vi "Convert Rx Config (4 Channels).vi"(0 "rx config":T2={"transfer mode"=enum."Finite", "sample rate"=10000000.0, "number of samples"=8192, "start trigger"=enum."Immediate", "daughterboard 0 config"={"rf enable 0"=TRUE, "rf config 0"={"antenna"="RX1", "frequency"=2000000000.0, "gain"=40.0}, "rf enable 1"=TRUE, "rf config 1"={"antenna"="RX2", "frequency"=2000000000.0, "gain"=40.0}, "lo configuration"=enum."Independent"}, "daughterboard 1 config"={"rf enable 2"=TRUE, "rf config 2"={"antenna"="RX1", "frequency"=2000000000.0, "gain"=40.0}, "rf enable 3"=TRUE, "rf config 3"={"antenna"="RX2", "frequency"=2000000000.0, "gain"=40.0}, "lo configuration"=enum."Independent"}} {"daughterboard 1 config"."rf config 3"."gain" format="%#.1f"; "daughterboard 1 config"."rf config 3"."frequency" format="%#.3pHz"; "daughterboard 1 config"."rf config 2"."gain" format="%#.1f"; "daughterboard 1 config"."rf config 2"."frequency" format="%#.3pHz"; "daughterboard 0 config"."rf config 1"."gain" format="%#.1f"; "daughterboard 0 config"."rf config 1"."frequency" format="%#.3pHz"; "daughterboard 0 config"."rf config 0"."gain" format="%#.1f"; "daughterboard 0 config"."rf config 0"."frequency" format="%#.3pHz"; "sample rate" format="%#.3pS/s"}) -> (4 "rx config out":T4={"channel configuration"=[], "transfer mode"=enum."Finite", "sample rate"=10000000.0, "number of samples"=8192, "start trigger"=enum."Immediate"} {"channel configuration"."channel configuration"."frequency" format="%#.3pHz"; "channel configuration"."channel configuration"."lo frequency" format="%#.3pHz"; "channel configuration"."channel configuration"."level" format="%#_gdBm"; "sample rate" format="%#.3pS/s"}, 6 "lo config out":T3)   [LabVIEW 2016]
uses:
  Start Trigger.ctl
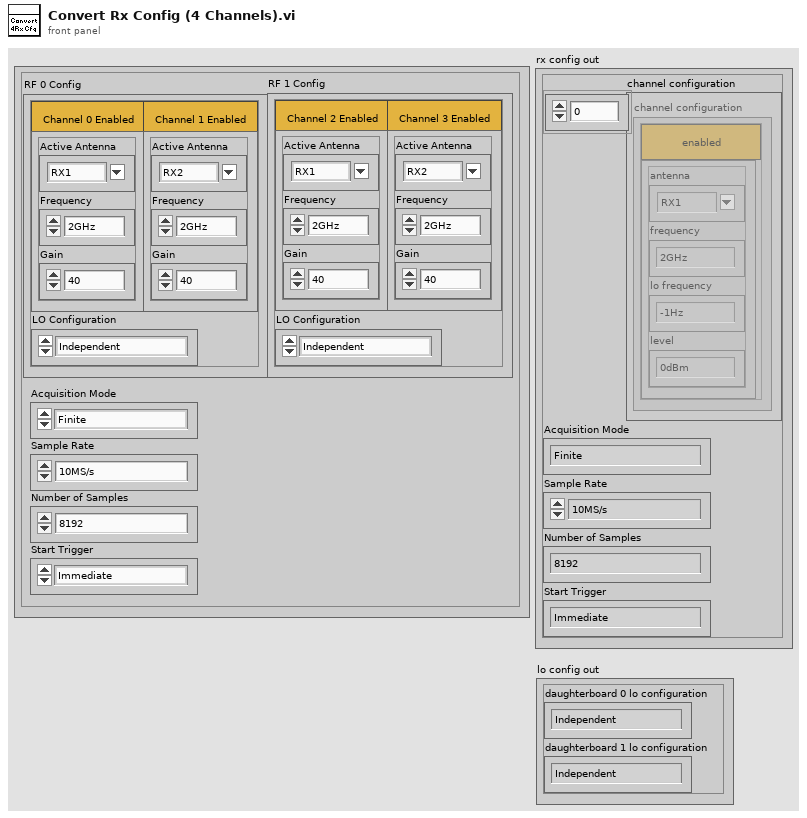
[diagram p1: front panel]
types:
  T1 = typedef "Start Trigger.ctl" = enum8{"Software", "Digital Edge", "Rx Start Trigger", "Tx Start Trigger", "Immediate", "Future Time Event"}
  T2 = cluster{"transfer mode":enum16{"Finite", "Continuous"}, "sample rate":dbl, "number of samples":u32, "start trigger":T1, "daughterboard 0 config":cluster{"rf enable 0":bool, "rf config 0":cluster{"antenna":string, "frequency":dbl, "gain":dbl}, "rf enable 1":bool, "rf config 1":cluster{"antenna":string, "frequency":dbl, "gain":dbl}, "lo configuration":enum16{"Independent", "Import"}}, "daughterboard 1 config":cluster{"rf enable 2":bool, "rf config 2":cluster{"antenna":string, "frequency":dbl, "gain":dbl}, "rf enable 3":bool, "rf config 3":cluster{"antenna":string, "frequency":dbl, "gain":dbl}, "lo configuration":enum16{"Independent", "Import", "Shared and Export"}}}
  T3 = cluster{"daughterboard 0 lo configuration":enum16{"Independent", "Import", "Shared and Export"}, "daughterboard 1 lo configuration":enum16{"Independent", "Import", "Shared and Export"}}
  T4 = cluster{"channel configuration":cluster{"channel enable":bool, "channel configuration":cluster{"antenna":string, "frequency":dbl, "lo frequency":dbl, "level":dbl}}[], "transfer mode":enum16{"Finite", "Continuous"}, "sample rate":dbl, "number of samples":u32, "start trigger":T1}
  T5 = cluster{"channel enable":bool, "channel configuration":cluster{"antenna":string, "frequency":dbl, "lo frequency":dbl, "level":dbl}}
  T6 = enum16{"Independent", "Import", "Shared and Export"}
  T7 = cluster{"channel enable":bool, "channel configuration":cluster{"antenna":string, "frequency":dbl, "lo frequency":dbl, "level":dbl}}[]
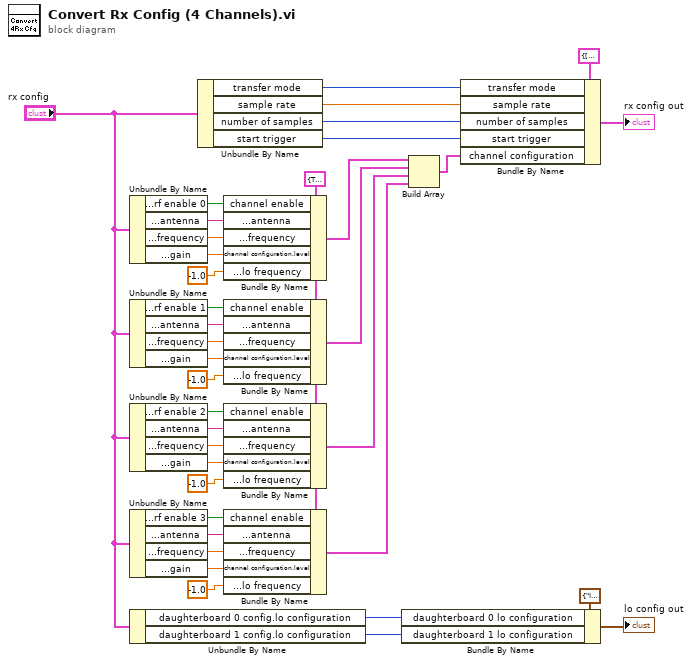
[diagram p0: block diagram]
diagram:
  w11 = T5 {"channel enable"=TRUE, "channel configuration"={"antenna"="RX1", "frequency"=2000000000.0, "lo frequency"=-1.0, "level"=0.0}} ("channel configuration")
  n1 = Unbundle By Name("rx config") -> ("daughterboard 0 config.rf enable 0"=w30:bool, "daughterboard 0 config.rf config 0.antenna"=w29:string, "daughterboard 0 config.rf config 0.frequency"=w28:dbl, "daughterboard 0 config.rf config 0.gain"=w27:dbl)
  n2 = Unbundle By Name("rx config") -> ("daughterboard 0 config.rf enable 1"=w26:bool, "daughterboard 0 config.rf config 1.antenna"=w25:string, "daughterboard 0 config.rf config 1.frequency"=w24:dbl, "daughterboard 0 config.rf config 1.gain"=w13:dbl)
  n3 = Unbundle By Name("rx config") -> ("daughterboard 1 config.rf enable 2"=w23:bool, "daughterboard 1 config.rf config 2.antenna"=w22:string, "daughterboard 1 config.rf config 2.frequency"=w21:dbl, "daughterboard 1 config.rf config 2.gain"=w20:dbl)
  n4 = Unbundle By Name("rx config") -> ("daughterboard 1 config.rf enable 3"=w19:bool, "daughterboard 1 config.rf config 3.antenna"=w18:string, "daughterboard 1 config.rf config 3.frequency"=w17:dbl, "daughterboard 1 config.rf config 3.gain"=w16:dbl)
  n5 = Unbundle By Name("rx config") -> ("daughterboard 0 config.lo configuration"=w5:enum16{"Independent", "Import"}, "daughterboard 1 config.lo configuration"=w4:T6)
  n6 = Unbundle By Name("rx config") -> ("transfer mode"=w37:enum16{"Finite", "Continuous"}, "sample rate"=w36:dbl, "number of samples"=w35:u32, "start trigger"=w34:T1)
  n7 = Bundle By Name(cluster=w11, "channel enable"=w30, "channel configuration.antenna"=w29, "channel configuration.frequency"=w28, "channel configuration.level"=w27, "channel configuration.lo frequency"=-1.0 ("lo frequency")) -> (w9:T5)
  n8 = Bundle By Name(cluster=w11, "channel enable"=w26, "channel configuration.antenna"=w25, "channel configuration.frequency"=w24, "channel configuration.level"=w13, "channel configuration.lo frequency"=-1.0 ("lo frequency")) -> (w8:T5)
  n9 = Bundle By Name(cluster=w11, "channel enable"=w23, "channel configuration.antenna"=w22, "channel configuration.frequency"=w21, "channel configuration.level"=w20, "channel configuration.lo frequency"=-1.0 ("lo frequency")) -> (w7:T5)
  n10 = Bundle By Name(cluster=w11, "channel enable"=w19, "channel configuration.antenna"=w18, "channel configuration.frequency"=w17, "channel configuration.level"=w16, "channel configuration.lo frequency"=-1.0 ("lo frequency")) -> (w6:T5)
  n11 = Bundle By Name(cluster=T3 {"daughterboard 0 lo configuration"=enum."Independent", "daughterboard 1 lo configuration"=enum."Independent"} ("lo config"), "daughterboard 0 lo configuration"=w5, "daughterboard 1 lo configuration"=w4) -> (→"lo config out":T3)
  n12 = Build Array(w9, w8, w7, w6) -> (w10:T7)
  n13 = Bundle By Name(cluster=T4 {"channel configuration"=[], "transfer mode"=enum."Finite", "sample rate"=10000000.0, "number of samples"=8192, "start trigger"=enum."Immediate"} ("rx config"), "transfer mode"=w37, "sample rate"=w36, "number of samples"=w35, "start trigger"=w34, "channel configuration"=w10) -> (→"rx config out":T4)
